vi "iscan.vi"(3 "Draw":enum16{"I(Ewe)", "Ewe(t)", "I(t)", "Test"}(ring)=enum."I(t)", 7 "DLLPath":path, 8 "error in (no error)":errorcluster, 9 "ISCAN Parameters":T2={"vs_initial "=TRUE, "Current_step"=0.0, "Scans"=[{" vs_initial"=FALSE, "Current_step"=0.001, "Scan_Rate"=1.0}, {" vs_initial"=FALSE, "Current_step"=-0.001, "Scan_Rate"=1.0}, {" vs_initial"=FALSE, "Current_step"=0.0, "Scan_Rate"=1.0}], "Scan_number"=2, "N_Cycles"=1, "Record_every_dI"=1e-05, "Begin_measuring_E"=0.5, "End_measuring_E"=0.75, "I_Range"=7, "E_Range"=2, "Bandwidth"=5, "em"=1, "ce"=0, "tb"=5e-05} {"tb" min=5e-05 max=1 format="%^_3e"; "ce" items=["Standard", "CE to ground"]; "End_measuring_E" min=0 max=1 format="%.2f"; "Begin_measuring_E" min=0 max=1 format="%.2f"; "Current_step" min=-150 max=150 format="%^_3e"; "N_Cycles" min=0 max=1000000; "Scan_number" min=0 max=98; "Scans"."Scan_Rate" min=0.01 max=1000 format="%^_3e"; "Scans"."Current_step" min=-150 max=150 format="%^_3e"; "E_Range" items=["±2.5V", "±5V", "±10V", "Auto"]; "Bandwidth" items=["1"=1, "2"=2, "3"=3, "4"=4, "5"=5, "6"=6, "7"=7, "8"=8, "9"=9]; "Record_every_dI" format="%^_3e"; "I_Range" items=["1pA", "1nA", "10nA", "100nA", "1µA", "10µA", "100µA", "1mA", "10mA", "100mA", "1A", "Booster"]}, 10 "Channel":u8(ring)=12 items=["1", "2", "3", "4", "5", "6", "7", "8", "9", "10", "11", "12", "13", "14", "15", "16"], 11 "IP adress":string="192.109.209.229") -> (0 "error out":errorcluster, 1 "Output_Data":T1, 2 "Exit 2":bool=TRUE, 4 "XY Graph":cluster{"Data 101":sgl[], "Data 101":sgl[]}(graph))   [LabVIEW 2022 SP3]
doc: "The Current scan technique (Galvanodynamic Technique) technique allows the user to perform galvanodynamic periods with different scan rates.\nIn general, in this VI, the first thing to do is to start by establishing the connection with the instrument defined by its IP adress, then load the firmware in the channel selected, get the information on the plugged channels, load protocol on a channel, start/stop the protocol, retreive data and draw the graph."
uses:
  Library/EClib Functions/ISCANParameters.ctl
  Library/EClib Functions/Parameters.ctl
  Library/EClib Functions/EClib functions.lvlib
panel:
  out "cycle index":i32[](array[numeric])
  in  "Display Parameters?":bool caption="Display Parameters"
  out "DllPath":path caption="DLL Path"
  out "LibVersion":string caption="DLL Version"
  out "Device Code":i32
  out "Number of points":i32=105
  out "Data 125":sgl[][](array[numeric])=[[0.003, 0.0019739384, 6.01559e-07, 0.002076381], [0.105000004, 0.012167796, 2.1901733e-06, 0.0117511805], [0.20700002, 0.022361653, 3.975648e-06, 0.021977918], [0.30900002, 0.03255551, 5.772186e-06, 0.032090176], [0.411, 0.042749364, 7.5965745e-06, 0.042278755], [0.513, 0.052943222, 9.43279e-06, 0.052619968], [0.615, 0.06313708, 1.1011484e-05, 0.06277039], [0.717, 0.07333094, 1.3262951e-05, 0.07292081], [0.81900007, 0.08352479, 1.5135982e-05, 0.082956746], [0.92, 0.09371865, 1.6970866e-05, 0.09329796], [1.146, 0.08352479, 1.50444275e-05, 0.083796255], [1.248, 0.07333094, 1.3190472e-05, 0.07337872], [1.35, 0.06313708, 1.1359403e-05, 0.06338094], [1.4510001, 0.052943222, 9.505447e-06, 0.053039722], [1.5530001, 0.042749364, 7.704897e-06, 0.042965624], [1.6550001, 0.03255551, 5.7821057e-06, 0.03273889], [1.7570001, 0.022361653, 3.9939605e-06, 0.02243583], [1.8590001, 0.012167796, 2.2004742e-06, 0.012209094], [1.9610001, 0.0019739384, 3.9210917e-07, 0.0019060377], [2.0630002, -0.008219917, -1.42999e-06, -0.007939104], [2.1650002, -0.018413773, -3.2925293e-06, -0.01812768], [2.2670002, -0.02860763, -5.1661327e-06, -0.028087301], [2.3690002, -0.038801484, -7.0229494e-06, -0.038695633], [2.4710002, -0.048995342, -8.872135e-06, -0.048960526], [2.5730002, -0.059189197, -1.0682789e-05, -0.059149105], [2.6750002, -0.069383055, -1.2368184e-05, -0.06929952], [2.7770002, -0.07957691, -1.4145845e-05, -0.079564415], [2.8790002, -0.089770764, -1.595784e-05, -0.08963852], [2.9810002, -0.09996462, -1.7746945e-05, -0.09997973], [3.0830002, -0.11015848, -1.9597086e-05, -0.11005383], [3.1840003, -0.120352335, -2.1420525e-05, -0.1202424], [3.2860003, -0.13054618, -2.3339331e-05, -0.13024017], [3.3880002, -0.14074004, -2.5181842e-05, -0.14054324], [3.4900002, -0.1509339, -2.7039614e-05, -0.15061733], [3.5920002, -0.16112776, -2.8866867e-05, -0.16069143], [3.6940002, -0.17132162, -3.0690302e-05, -0.17118528], [3.7960002, -0.18151547, -3.246415e-05, -0.18129754], [3.8980002, -0.19170932, -3.425326e-05, -0.19167691], [4.1660004, -0.18151547, -3.2410746e-05, -0.1819081], [4.268, -0.17132162, -3.064834e-05, -0.17160504], [4.3700004, -0.16112776, -2.8840164e-05, -0.1615691], [4.472, -0.1509339, -2.6993837e-05, -0.15141869], [4.5740004, -0.14074004, -2.5170399e-05, -0.14126827], [4.676, -0.13054618, -2.3297369e-05, -0.13085073], [4.7780004, -0.120352335, -2.1454858e-05, -0.120471366], [4.88, -0.11015848, -1.9608531e-05, -0.11066438], [4.9820004, -0.09996462, -1.7731685e-05, -0.100361325], [5.084, -0.089770764, -1.5908246e-05, -0.09028722], [5.1860003, -0.07957691, -1.4138216e-05, -0.07979337], [5.288, -0.069383055, -1.23643695e-05, -0.06975743], [5.3900003, -0.059189197, -1.0510413e-05, -0.059530698], [5.491, -0.048995342, -8.728937e-06, -0.049342122], [5.5930004, -0.038801484, -6.897869e-06, -0.039191704], [5.695, -0.02860763, -5.1615543e-06, -0.029041288], [5.7970004, -0.018413773, -3.292148e-06, -0.018547434], [5.899, -0.008219917, -1.4265564e-06, -0.008549656], [6.0010004, 0.0019739384, 4.397981e-07, 0.0014481241], [6.103, 0.012167796, 2.245111e-06, 0.011636702], [6.2050004, 0.022361653, 4.0595805e-06, 0.021939758], [6.307, 0.03255551, 5.846962e-06, 0.032090176], [6.4090004, 0.042749364, 7.638159e-06, 0.04212612], [6.511, 0.052943222, 9.431646e-06, 0.05246733], [6.6130004, 0.06313708, 1.1045057e-05, 0.062579595], [6.715, 0.07333094, 1.3209546e-05, 0.07276817], [6.8170004, 0.08352479, 1.5067316e-05, 0.08303307], [6.919, 0.09371865, 1.690983e-05, 0.09318349], [7.1440005, 0.08352479, 1.5128351e-05, 0.08364362], [7.2460003, 0.07333094, 1.3301099e-05, 0.0733024], [7.3480005, 0.06313708, 1.1408995e-05, 0.06338094], [7.4490004, 0.052943222, 9.520706e-06, 0.053039726], [7.5510006, 0.042749364, 7.704897e-06, 0.042316914], [7.6530004, 0.03255551, 5.7290754e-06, 0.032624412], [7.7550006, 0.022361653, 3.9203287e-06, 0.02262663], [7.8570004, 0.012167796, 2.1073854e-06, 0.012056456], [7.9590006, 0.0019739384, 3.3221184e-07, 0.0022876323], [8.061001, -0.008219917, -1.4410538e-06, -0.007900944], [8.163, -0.018413773, -3.2478924e-06, -0.017975042], [8.265, -0.02860763, -5.089448e-06, -0.028316258], [8.367001, -0.038801484, -6.929479e-06, -0.038504835], [8.469001, -0.048995342, -8.814146e-06, -0.04869341], [8.571, -0.059189197, -1.0662569e-05, -0.059263583], [8.673, -0.069383055, -1.2417775e-05, -0.06933768], [8.775001, -0.07957691, -1.42297695e-05, -0.079144664], [8.877001, -0.089770764, -1.6053207e-05, -0.0893714], [8.979, -0.09996462, -1.7861388e-05, -0.09982709], [9.081, -0.11015848, -1.9642863e-05, -0.10990119], [9.182, -0.120352335, -2.1462487e-05, -0.12020425], [9.284, -0.13054618, -2.3247778e-05, -0.13043097], [9.386001, -0.14074004, -2.5071215e-05, -0.14046691], [9.488001, -0.1509339, -2.6944244e-05, -0.15084629], [9.59, -0.16112776, -2.8832534e-05, -0.16084407], [9.692, -0.17132162, -3.0682673e-05, -0.17129977], [9.794001, -0.18151547, -3.2525186e-05, -0.18110675], [9.896001, -0.19170932, -3.435244e-05, -0.19156244], [10.1640005, -0.18151547, -3.2357337e-05, -0.18206073], [10.266001, -0.17132162, -3.0552972e-05, -0.1716432], [10.368, -0.16112776, -2.8763869e-05, -0.16137831], [10.47, -0.1509339, -2.6936617e-05, -0.15138052], [10.5720005, -0.14074004, -2.5143696e-05, -0.14138275], [10.674001, -0.13054618, -2.3377479e-05, -0.1306981], [10.776001, -0.120352335, -2.1515893e-05, -0.12066216], [10.878, -0.11015848, -1.9719157e-05, -0.11047359], [10.9800005, -0.09996462, -1.780798e-05, -0.100513965], [11.082001, -0.089770764, -1.5946394e-05, -0.09021091], [11.184001, -0.07957691, -1.4088625e-05, -0.079869695]] format="%.2f"
  in  "stop":bool
  in  "Exit":bool
  in  "Start":bool
  # "Instructions:\nBefore running the VI you must type a valid IP adress that corresponds to the instrument.Then press the Run button to execute this VI.\nWhile this VI is running, choose the available channel, enter the ISCAN parameters or keep the default values, then press the button start to begin the experience.\nChoose the waveform to draw (Ewe(t) or I(t) or I(Ewe) or Ec(t). You can stop the measure if you press the stop button and exit the execution if you press the exit button."
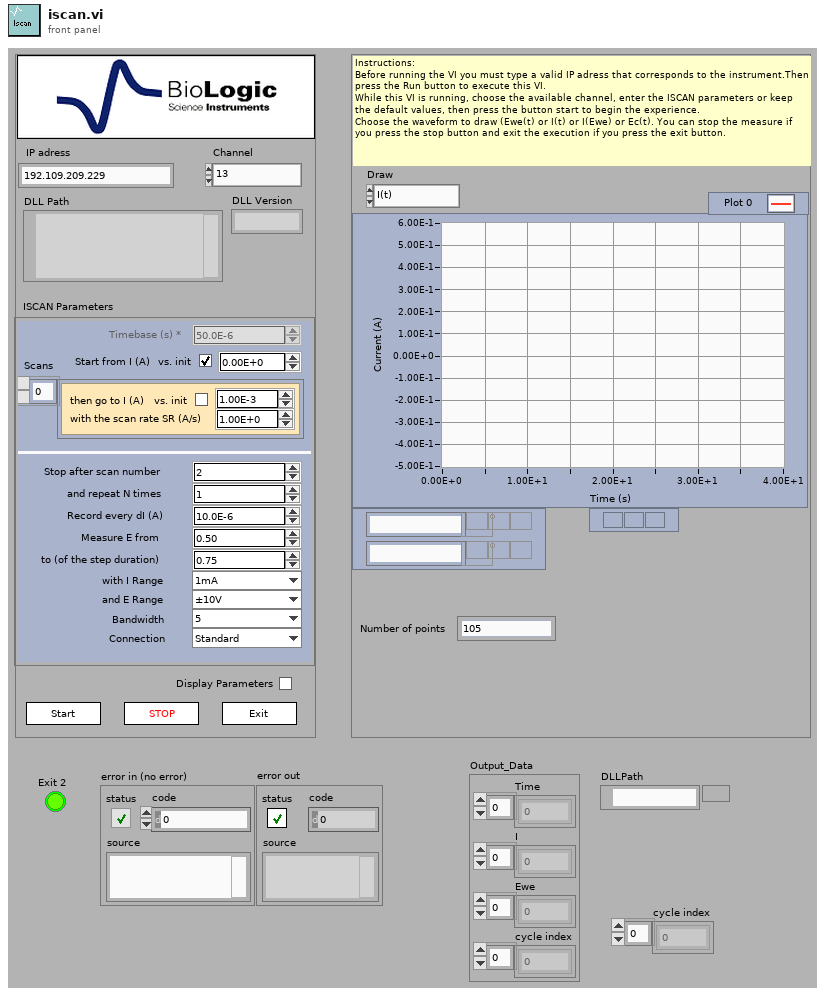
[diagram p1: front panel]
types:
  T1 = cluster{"Time":sgl[], "I":sgl[], "Ewe":sgl[], "cycle index":i32[]}
  T2 = typedef "EClib functions.lvlib/ISCANParameters.ctl" = cluster{"vs_initial ":bool, "Current_step":sgl, "Scans":cluster{" vs_initial":bool, "Current_step":sgl, "Scan_Rate":sgl}[], "Scan_number":i32, "N_Cycles":i32, "Record_every_dI":sgl, "Begin_measuring_E":sgl, "End_measuring_E":sgl, "I_Range":u16, "E_Range":u16, "Bandwidth":u16, "em":u16, "ce":u16, "tb":sgl}
  T3 = cluster{"LibVersion":string, "StringLength":u32, "DllPath":path}
  T4 = cluster{"Channel":i32, "BoardVersion":i32, "BoardSerialCode":i32, "FirmwareCode":i32, "FirmwareVersion":i32, "XilinxVersion":i32, "AmpCode":i32, "NbAmp":i32, "LcBoard":i32, "Zboard":i32, "MuxBoard":i32, "GPRAboard":i32, "MemSize":i32, "MemFilled":i32, "state":i32, "MaxIRange":i32, "MinIRange":i32, "MaxBandwidth":i32, "NbOfTechniques":i32}
  T5 = typedef "EClib functions.lvlib/Parameters.ctl" = enum16{"CA", "CASG", "CP", "GEIS", "ISCAN", "OCV", "PEIS", "SCCX", "SGEIS", "SPEIS", "VSCAN", "MP"}
  T6 = typedef "EClib functions.lvlib/TechniqueParameters.ctl" = cluster{"String Label":string, "Type":i32, "Valeur":i32, "Index":i32}
  T7 = cluster{"string before end tag":string, i32, i32, i32}[]
  T8 = cluster{"IRQskipped":i32, "NbRaws":i32, "NbCols":i32, "Technique Index":i32, "TechniqueID":i32, "PrcessIndex":i32, "loop":i32, "StartTime":dbl, "MuxPad":i32}
  T9 = cluster{"State":i32, "MemFilled":i32, "TimeBase":sgl, " Ewe":sgl, " EweRangeMin":sgl, " EweRangeMax":sgl, "Ece":sgl, "EceRangeMin":sgl, "EceRangeMax":sgl, "Eoverflow":i32, "I":sgl, "IRange":i32, "Ioverflow":i32, "ElapsedTime":sgl, "Freq":sgl, "Rcomp":sgl, "Saturation":sgl, "OptErr":i32, "OptPos":i32}
  T10 = cluster{"Data 125":sgl[], "Data 125":sgl[], "Data 125":sgl[], "cycle index":i32[]}
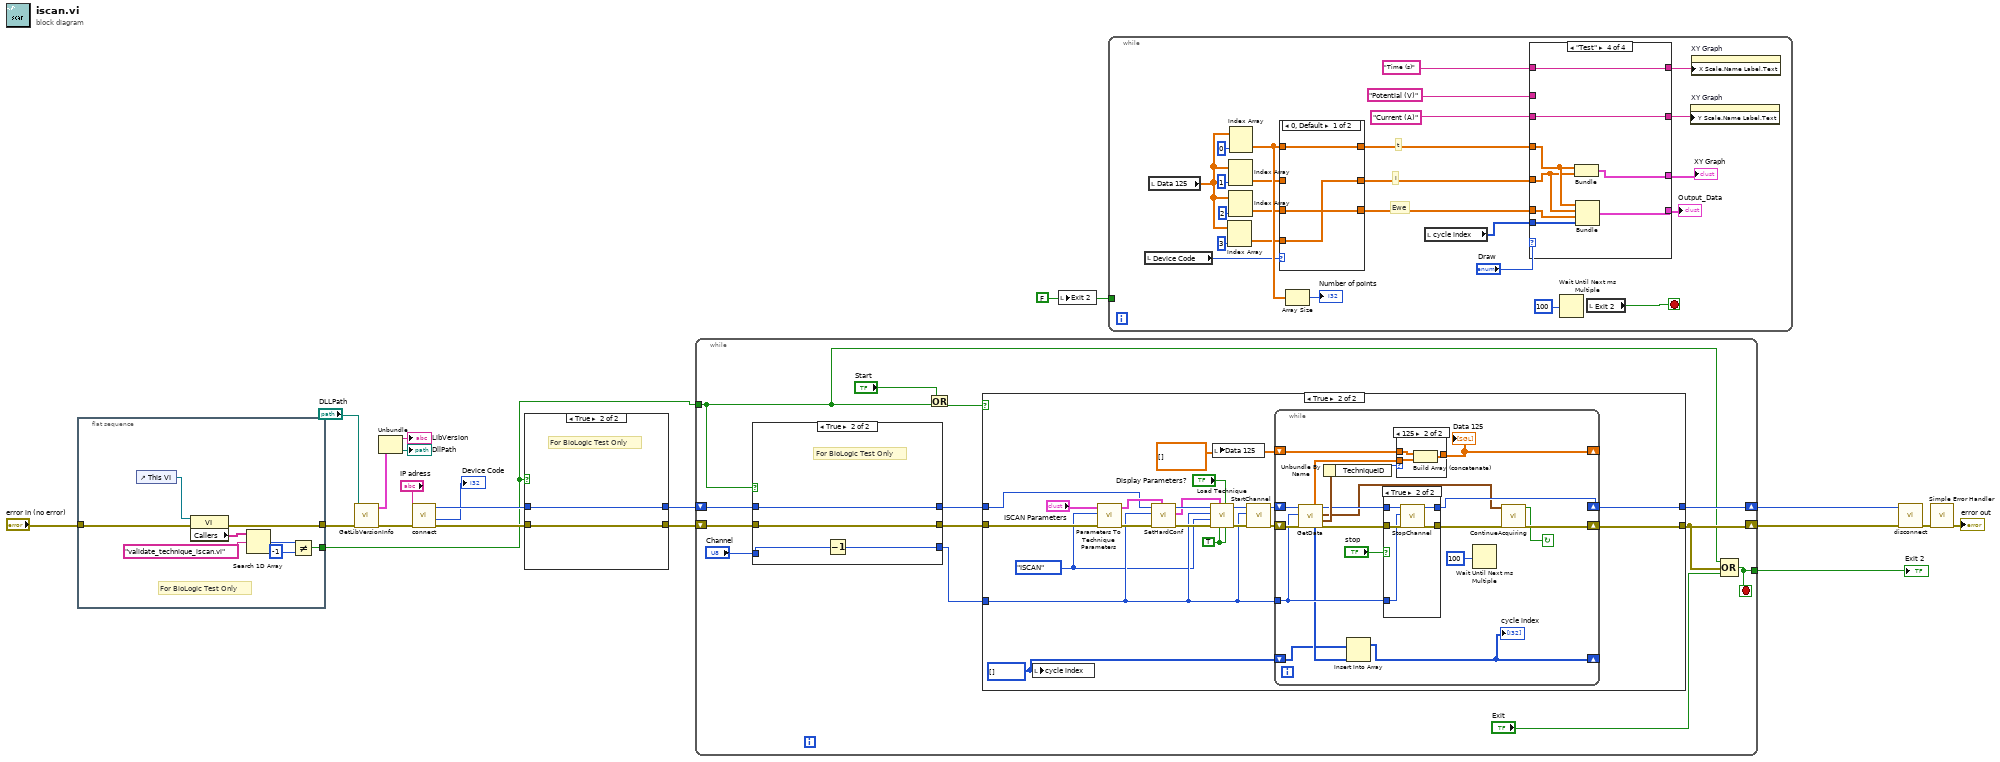
[diagram p0: block diagram]
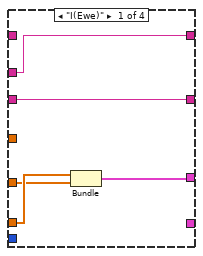
[diagram p3: hidden frame]
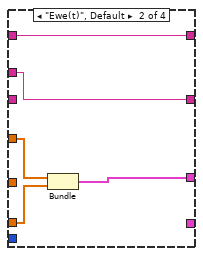
[diagram p4: hidden frame]
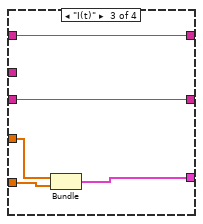
[diagram p5: hidden frame]
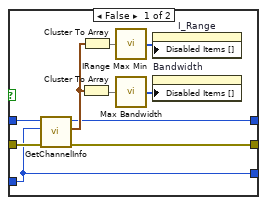
[diagram p9: hidden frame]
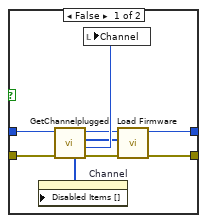
[diagram p10: hidden frame]
diagram:
  w20 = FALSE ("Exit 2")
  n1 = flat-sequence {
    tunnel: "error in (no error)" -> [w27]
    tunnel: [w26] -> w5
    tunnel: [w21] -> w2
    frame #0 {
      # "For BioLogic Test Only"
      n2 = control-ref of="This VI"() -> (w28:refnum<vi>)
      n3 = property class="VI"(reference=w28, error in=w27) -> (error out=w26:errorcluster, "Callers"=w25:string[])  [unwired: 1 out]
      n4 = Search 1D Array(1D array=w25, element="validate_technique_iscan.vi") -> (index of element=w23:i32)  [unwired: 1 in]
      n5 = Not Equal?(x=w23, y=-1) -> (x != y?=w21:bool)
    }
  }
  n6 = call "GetLibVersionInfo.vi"("error in (no error)"=w5, "DLLPath"="DLLPath") -> ("error out"=w7:errorcluster, "LibInfo"=w10:T3)  [unwired: 8 in]
  n7 = Unbundle(w10) -> ("LibVersion"=→"LibVersion":string, "DllPath"=→"DllPath":path)  [unwired: 1 out]
  n8 = call "connect.vi"("error in (no error)"=w7, "IP"="IP adress") -> ("error out"=w17:errorcluster, "Device Code"=→"Device Code":i32, "ID Out"=w18:i32)  [unwired: 5 in, 2 out]
  n9 = case shown="True" w2 {
    tunnel: w18 -> [w35 w38]
    tunnel: w17 -> [w34 w37]
    tunnel: [w30 w37] -> w16
    tunnel: [w29 w38] -> w6
    frame False {
      n10 = call "GetChannelplugged.vi"("error in (no error)"=w34, "ID In"=w35) -> ("error out"=w33:errorcluster, "FirstPluggedChannel"=w36:u8, "PluggedChannels"=w31:u8[], "DisabledChannels"=w32:i32[])  [unwired: 5 in, 1 out]
      n11 = property on="Channel" class="Ring (strict)"("Disabled Items []"=w32) -> ()  [unwired: 2 in, 2 out]
      n12 = local write "Channel"(w36) -> ()
      n13 = call "Load Firmware.vi"("error in (no error)"=w33, "Channels"=w31, "ID In"=w35) -> ("error out"=w30:errorcluster, "ID Out"=w29:i32)  [unwired: 6 in, 1 out]
    }
    frame True {
      # "For BioLogic Test Only"
    }
  }
  n14 = while {
    shift-right: [w46] -> w15
    shift-left: w16 -> [w49]
    shift-right: [w47] -> w13
    shift-left: w6 -> [w50]
    tunnel: [w44] -> w12
    tunnel: w2 -> [w39]
    stop <- w44 stop-if-true
    n15 = case shown="True" w39 {
      tunnel: w50 -> [w110 w118]
      tunnel: w49 -> [w109 w117]
      tunnel: "Channel" -> [w105 w116]
      tunnel: [w108 w117] -> w42
      tunnel: [w106 w118] -> w41
      tunnel: [w105 w115] -> w43
      frame False {
        n16 = call "GetChannelInfo.vi"("error in (no error)"=w109, "Channel"=w105, "ID"=w110) -> ("error out"=w108:errorcluster, "Channel information"=w107:T4, "ID Out"=w106:i32)  [unwired: 6 in]
        n17 = Cluster To Array(cluster=w107) -> (array=w113:i32[])
        n18 = Cluster To Array(cluster=w107) -> (array=w114:i32[])
        n19 = call "IRange Max Min.vi"("resources"=w114) -> ("disabled ranges"=w111:i32[])
        n20 = call "Max Bandwidth.vi"("resources"=w113) -> ("disabled ranges"=w112:i32[])
        n21 = property on="I_Range" class="Ring (strict)"("Disabled Items []"=w111) -> ()  [unwired: 2 in, 2 out]
        n22 = property on="Bandwidth" class="Ring (strict)"("Disabled Items []"=w112) -> ()  [unwired: 2 in, 2 out]
      }
      frame True {
        # "For BioLogic Test Only"
        n23 = Decrement(x=w116) -> (x-1=w115:u8)
      }
    }
    n24 = Or(x="Start", y=w39) -> (x .or. y?=w40:bool)
    n25 = case shown="True" w40 {
      tunnel: w43 -> [_ w57]
      tunnel: [w53 w73] -> w46
      tunnel: w42 -> [w53 w58]
      tunnel: [w52 w65] -> w47
      tunnel: w41 -> [w52 w56]
      frame False {
      }
      frame True {
        w54 = i32[] [] ("cycle index")
        w55 = Parameters."ISCAN" ("Parameters")
        w70 = TRUE ("First Protocol")
        w72 = sgl[][] []
        n26 = local write "cycle index"(w54) -> ()
        n27 = call "Parameters To Technique Parameters.vi"("error in (no error)"=w58, "Parameters"=w55, "ParameterIN"="ISCAN Parameters") -> ("error out"=w64:errorcluster, "Params Values"=w61:T6[])  [unwired: 7 in]
        n28 = call "SetHardConf.vi"("Params Values"=w61, "error in (no error)"=w64, "Channel"=w57, "ID In"=w56) -> ("error out"=w60:errorcluster, "Params Values Trimed"=w62:T7, "ID Out"=w63:i32)  [unwired: 5 in]
        n29 = call "Load Technique.vi"("Last Protocol"=w70, "Display Parameters?"="Display Parameters?", "First Protocol"=w70, "TechniqueParameters"=w62, "error in (no error)"=w60, "Parameters"=w55, "Selected Channel"=w57, "ID In"=w63) -> ("error out"=w69:errorcluster, "ID  Out"=w68:i32)  [unwired: 1 in, 1 out]
        n30 = local write "Data 125"(w72) -> ()
        n31 = call "StartChannel.vi"("error in (no error)"=w69, "Channel"=w57, "ID In"=w68) -> ("error out"=w67:errorcluster, "ID Out"=w66:i32)  [unwired: 7 in]
        n32 = while {
          shift-right: [w79] -> w73
          shift-left: w67 -> [w93]
          shift-right: [w90] -> _
          shift-left: w72 -> [w91]
          shift-right: [w82] -> w65
          shift-left: w66 -> [w85]
          tunnel: w57 -> [w81]
          shift-right: [w76] -> _
          shift-left: w54 -> [w74]
          stop <- w77 continue-if-true
          n33 = call "GetData.vi"("error in (no error)"=w93, "Channel"=w81, "ID In"=w85) -> ("error out"=w84:errorcluster, "Data information"=w87:T8, "Current values"=w80:T9, "ID Out"=w83:i32, "row2"=w75:u32[], "Data"=w86:dbl[][])  [unwired: 1 in, 2 out]
          n34 = Unbundle By Name(w87) -> ("TechniqueID"=w88:i32)
          n35 = Insert Into Array(array=w74, new element=w75) -> (w76:i32[])  [unwired: 1 in]
          "cycle index" <- w76
          n36 = case shown="True" "stop" {
            tunnel: [w94 w100] -> w78
            tunnel: w84 -> [w94 w99]
            tunnel: w83 -> [w95 w98]
            tunnel: [w95 w97] -> w82
            tunnel: w81 -> [_ w96]
            frame False {
            }
            frame True {
              n37 = call "StopChannel.vi"("error in (no error)"=w99, "Channel"=w96, "ID In"=w98) -> ("error out"=w100:errorcluster, "ID Out"=w97:i32)  [unwired: 7 in]
            }
          }
          n38 = case shown="125" w88 {
            tunnel: w91 -> [w101 w104]
            tunnel: [w101 w103] -> w90
            tunnel: w86 -> [_ w102]
            frame 0, Default {
            }
            frame 125 {
              n39 = Build Array (concatenate)(w104, w102) -> (w103:dbl[][])
            }
          }
          "Data 125" <- w90
          n40 = Wait Until Next ms Multiple(millisecond multiple=u32 100) -> ()  [unwired: 1 out]
          n41 = call "ContinueAcquiring.vi"("error in"=w78, "Current values"=w80) -> ("error out"=w79:errorcluster, "ContinueAcquiring?"=w77:bool)  [unwired: 8 in]
        }
      }
    }
    n42 = Compound Arithmetic op=OR(w39, w46, "Exit") -> (w44:bool)
  }
  "Exit 2" <- w12
  n43 = local write "Exit 2"(w20) -> ()
  n44 = while {
    tunnel: w20 -> [_]
    stop <- w142 stop-if-true
    # "Ewe"
    # "I"
    # "t"
    n45 = local read "Device Code"() -> (w121:i32)
    n46 = local read "Data 125"() -> (w130:sgl[][])
    n47 = Index Array(array=w130, index (col)=3 ("Index")) -> (element=w123:sgl[])  [unwired: 1 in]
    n48 = Index Array(array=w130, index (col)=1 ("Index")) -> (element=w126:sgl[])  [unwired: 1 in]
    n49 = Index Array(array=w130, index (col)=2 ("Index")) -> (element=w125:sgl[])  [unwired: 1 in]
    n50 = Index Array(array=w130, index (col)=0 ("Index")) -> (element=w128:sgl[])  [unwired: 1 in]
    n51 = case shown="0, Default" w121 {
      tunnel: w128 -> [w146 w149]
      tunnel: [w146 w149] -> w127
      tunnel: w126 -> [_ w148]
      tunnel: w125 -> [w145 w147]
      tunnel: [w145 w148] -> w124
      tunnel: w123 -> [w144 _]
      tunnel: [w144 w147] -> w122
      frame 0, Default {
      }
      frame 12, 16, 20, 21, 23, 27 {
      }
    }
    n52 = Array Size(array=w128) -> (size(s)=→"Number of points":i32)
    n53 = local read "cycle index"() -> (w119:i32[])
    n54 = case shown="\"Test\"" "Draw" {
      tunnel: w127 -> [_ w159 w164 w169]
      tunnel: w124 -> [w151 _ w163 w168]
      tunnel: [w150 w155 w160 w170] -> w129
      tunnel: "Potential (V)" ("Y Scale.Name Label.Text") -> [w154 w158 _ _]
      tunnel: "Current (A)" ("Y Scale.Name Label.Text") -> [w153 _ w162 w171]
      tunnel: [w153 w158 w162 w171] -> w134
      tunnel: [w154 w157 w161 w172] -> w133
      tunnel: "Time (s)" ("Y Scale.Name Label.Text") -> [_ w157 w161 w172]
      tunnel: w122 -> [w152 w156 _ w167]
      tunnel: [_ _ _ w166] -> w120
      tunnel: w119 -> [_ _ _ w165]
      frame "I(Ewe)" {
        n55 = Bundle("Data 125"=w152, "Data 125"=w151) -> (w150:cluster{"Data 125":sgl[], "Data 125":sgl[]})  [unwired: 1 in]
      }
      frame "Ewe(t)", Default {
        n56 = Bundle("Data 125"=w159, "Data 125"=w156) -> (w155:cluster{"Data 125":sgl[], "Data 125":sgl[]})  [unwired: 1 in]
      }
      frame "I(t)" {
        n57 = Bundle("Data 125"=w164, "Data 125"=w163) -> (w160:cluster{"Data 125":sgl[], "Data 125":sgl[]})  [unwired: 1 in]
      }
      frame "Test" {
        n58 = Bundle("Data 125"=w169, "Data 125"=w168) -> (w170:cluster{"Data 125":sgl[], "Data 125":sgl[]})  [unwired: 1 in]
        n59 = Bundle("Data 125"=w169, "Data 125"=w168, "Data 125"=w167, "cycle index"=w165) -> (w166:T10)  [unwired: 1 in]
      }
    }
    "XY Graph" <- w129
    "Output_Data" <- w120
    n60 = Wait Until Next ms Multiple(millisecond multiple=u32 100) -> ()  [unwired: 1 out]
    n61 = local read "Exit 2"() -> (w142:bool)
    n62 = property on="XY Graph" class="XYGraph (strict)"("Y Scale.Name Label.Text"=w134) -> ()  [unwired: 2 in, 2 out]
    n63 = property on="XY Graph" class="XYGraph (strict)"("X Scale.Name Label.Text"=w133) -> ()  [unwired: 2 in, 2 out]
  }
  n64 = call "disconnect.vi"("error in (no error)"=w15, "ID In"=w13) -> ("error out"=w11:errorcluster)  [unwired: 9 in]
  n65 = call <vilib>:"Simple Error Handler.vi"("error in (no error)"=w11) -> ("error out"=→"error out":errorcluster)  [unwired: 4 in, 4 out]
